vi "Del ExpGroup.vi"(8 "error in (no error)":errorcluster, 11 "Control-Client in":refnum<class "Control-Client.lvclass">) -> (0 "error out":errorcluster, 3 "Control-Client out":refnum<class "Control-Client.lvclass">)   [LabVIEW 2015, in "Control-Client.lvclass"]
uses:
  Control-Client.lvclass
  Control-Client.lvclass/Control-Client.ctl
  Experiments/Experiments_group.lvclass
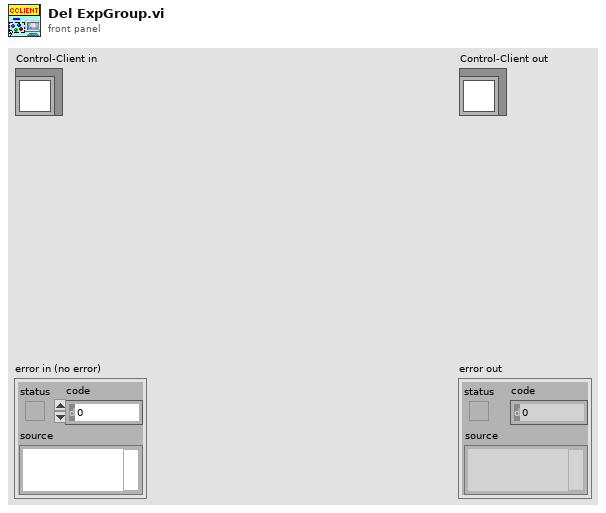
[diagram p1: front panel]
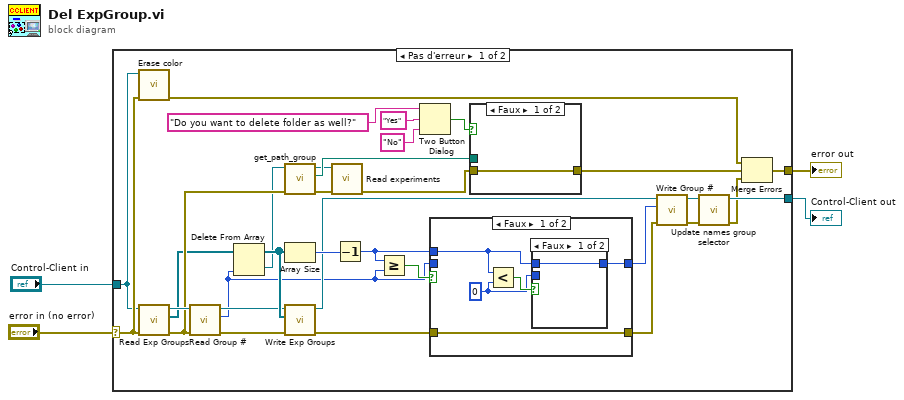
[diagram p0: block diagram]
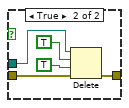
[diagram p4: hidden frame]
diagram:
  n1 = case shown="Pas d'erreur" "error in (no error)" {
    selector: "error in (no error)" -> [w9 w53]
    tunnel: [w19 w53] -> w3
    tunnel: [w28 w52] -> w1
    tunnel: "Control-Client in" -> [w8 w52]
    frame No Error {
      n2 = call "Erase color.vi"("error in (no error)"=w9, "Control-Client in"=w8) -> ("error out"=w7:errorcluster)  [unwired: 8 in, 1 out]
      n3 = call "Read Exp Groups.vi"("error in (no error)"=w9, "Control-Client in"=w8) -> ("error out"=w24:errorcluster, "Exp Groups"=w6:refnum<class "Experiments_group.lvclass">[], "Control-Client out"=w32:refnum<class "Control-Client.lvclass">)  [unwired: 7 in]
      n4 = call "Read Group #.vi"("error in (no error)"=w24, "Control-Client in"=w32) -> ("error out"=w27:errorcluster, "Group #"=w5:i32, "Control-Client out"=w26:refnum<class "Control-Client.lvclass">)  [unwired: 7 in]
      n5 = Delete From Array(array=w6, index=w5) -> (deleted portion=w23:refnum<class "Experiments_group.lvclass">, array with subset deleted=w30:refnum<class "Experiments_group.lvclass">[])  [unwired: 1 in]
      n6 = call "get_path_group.vi"("error in (no error)"=w24, "Experiments_group.lvclass in"=w23) -> ("error out"=w13:errorcluster, "Path"=w22:path, "Experiments_group.lvclass out"=w14:refnum<class "Experiments_group.lvclass">)  [unwired: 7 in]
      n7 = Array Size(array=w30) -> (size(s)=w25:i32)
      n8 = call "Write Exp Groups.vi"("error in (no error)"=w27, "Exp Groups"=w30, "Control-Client in"=w26) -> ("error out"=w10:errorcluster, "Control-Client out"=w11:refnum<class "Control-Client.lvclass">)  [unwired: 7 in]
      n9 = call "Read experiments.vi"("error in (no error)"=w13, "Experiments_group.lvclass in"=w14) -> ("error out"=w12:errorcluster)  [unwired: 6 in, 2 out]
      n10 = Decrement(x=w25) -> (x-1=w16:i32)
      n11 = Greater Or Equal?(x=w16, y=w5) -> (x >= y?=w18:bool)
      n12 = Two Button Dialog(message="Do you want to delete folder as well?", 1:"No" ("F button name (\"Cancel\")"), 2:"Yes" ("T button name (\"OK\")")) -> (T button?=w33:bool)
      n13 = case shown="Faux" w18 {
        tunnel: [w39 w45] -> w17
        tunnel: w5 -> [_ w45]
        tunnel: w16 -> [w37 _]
        tunnel: w10 -> [w41 w44]
        tunnel: [w41 w44] -> w15
        frame False {
          w38 = 0 ("y")
          n14 = Less?(x=w37, y=w38) -> (x < y?=w40:bool)
          n15 = case shown="Faux" w40 {
            tunnel: [w42 w43] -> w39
            tunnel: w38 -> [_ w43]
            tunnel: w37 -> [w42 _]
            frame False {
            }
            frame True {
            }
          }
        }
        frame True {
        }
      }
      n16 = case shown="Faux" w33 {
        tunnel: w22 -> [_ w49]
        tunnel: w12 -> [w46 w48]
        tunnel: [w46 w47] -> w21
        frame False {
        }
        frame True {
          n17 = Delete(path (use dialog)=w49, entire hierarchy (F)=TRUE, confirm (F)=TRUE, error in=w48) -> (error out=w47:errorcluster)  [unwired: 1 in, 2 out]
        }
      }
      n18 = call "Write Group #.vi"("error in (no error)"=w15, "Group #"=w17, "Control-Client in"=w11) -> ("error out"=w31:errorcluster, "Control-Client out"=w29:refnum<class "Control-Client.lvclass">)  [unwired: 7 in]
      n19 = call "Update names group selector.vi"("error in (no error)"=w31, "Control-Client in"=w29) -> ("error out"=w20:errorcluster, "Control-Client out"=w28:refnum<class "Control-Client.lvclass">)  [unwired: 8 in]
      n20 = Merge Errors(w7, w21, w20) -> (w19:errorcluster)
    }
    frame Error {
    }
  }
  "error out" <- w3
  "Control-Client out" <- w1
